vi "TEMPDo.vi"(8 "error in (no error)":errorcluster, 10 "Actor in":refnum<class "Actor.lvclass">, 11 "DNL_Message Template":refnum<class "Message.lvclass">) -> (0 "error out":errorcluster, 2 "Actor out":refnum<class "Actor.lvclass">)   [LabVIEW 2016, in "AsynchReturn Template.lvclass"]
doc: "This VI delivers the message to the actor by calling the appropriate method(s) on the actor."
uses:
  AsynchReturn Template.lvclass
  <vilib>/ActorFramework/Actor/Actor.lvclass
  <vilib>/ActorFramework/Message/Message.lvclass
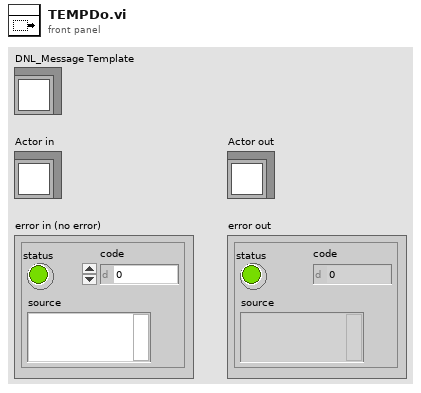
[diagram p1: front panel]
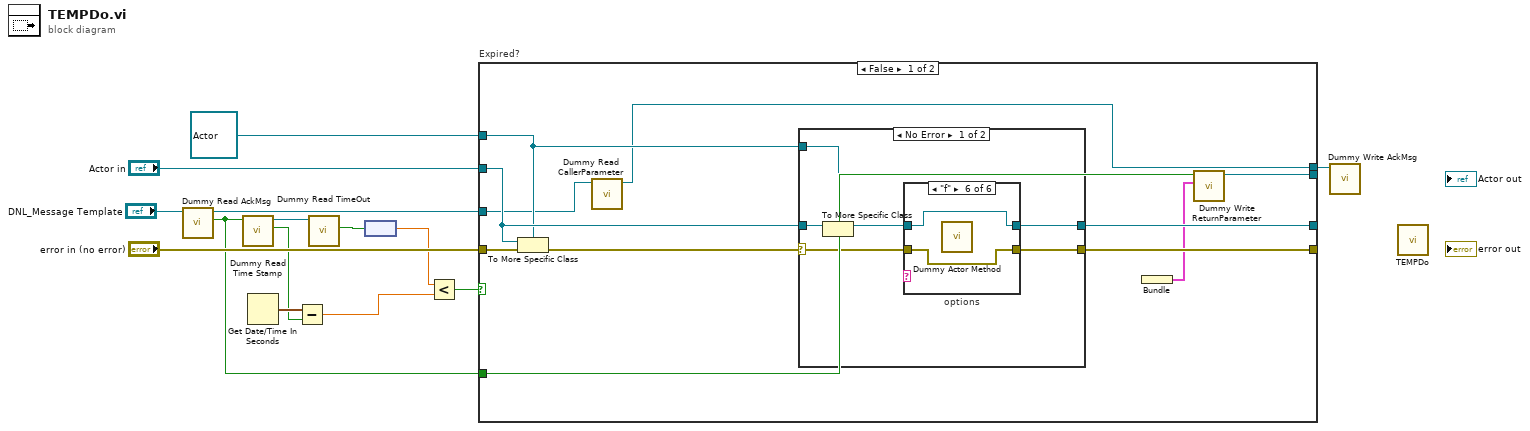
[diagram p0: block diagram]
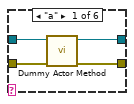
[diagram p2: hidden frame]
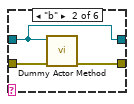
[diagram p3: hidden frame]
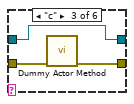
[diagram p4: hidden frame]
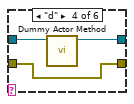
[diagram p5: hidden frame]
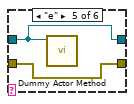
[diagram p6: hidden frame]
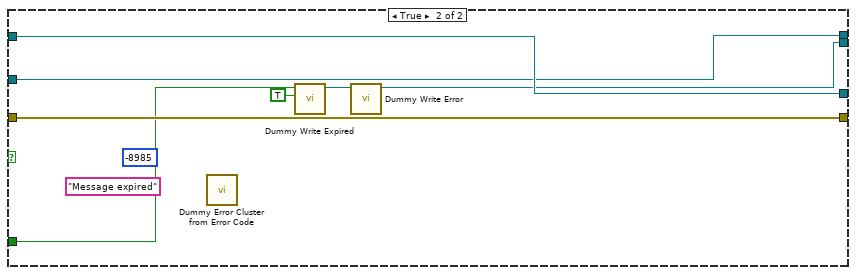
[diagram p8: hidden frame]
diagram:
  n1 = call "Dummy Read AckMsg.vi"("Actor in"="DNL_Message Template") -> ("Boolean"=w2:bool, "Actor out"=w3:refnum<class "Actor.lvclass">)  [unwired: 8 in, 1 out]
  n2 = call "Dummy Read Time Stamp.vi"("Actor in"=w2) -> ("Boolean"=w9:bool, "Actor out"=w8:refnum<class "Actor.lvclass">)  [unwired: 8 in, 1 out]
  n3 = Get Date/Time In Seconds() -> (seconds since 1Jan1904=w10:timestamp)
  n4 = Subtract(x=w10, y=w9) -> (x-y=w5:dbl)
  n5 = call "Dummy Read TimeOut.vi"("Actor in"=w8) -> ("Boolean"=w7:bool)  [unwired: 8 in, 2 out]
  n6 = node(w7) -> (w6:dbl[unit])
  n7 = Less?(x=w6, y=w5) -> (x < y?=w4:bool)
  n8 = case "Expired?" shown="False" w4 {
    tunnel: [w25 w56] -> _
    tunnel: [w24 w57] -> _
    tunnel: "Actor in" -> [w23 w57]
    tunnel: refnum<class "Actor.lvclass"> refnum ("Actor in") -> [w22 _]
    tunnel: "error in (no error)" -> [w21 w56]
    tunnel: w3 -> [w20 w52]
    tunnel: [w17 w52] -> w1
    tunnel: w2 -> [w18 w53]
    tunnel: [w16 w51] -> _
    frame False {
      n9 = To More Specific Class(target class=w22, reference=w23, error in=w21) -> (error out=w15:errorcluster)  [unwired: 1 out]
      n10 = call "Dummy Read CallerParameter.vi"("Actor in"=w20) -> ("Actor out"=w17:refnum<class "Actor.lvclass">)  [unwired: 8 in, 2 out]
      n11 = case "Error Case" shown="No Error" w15 {
        selector: w15 -> [w29 w50]
        tunnel: [w31 w50] -> w25
        tunnel: [w30 w49] -> w24
        tunnel: w23 -> [w28 w49]
        tunnel: w22 -> [w27 _]
        frame No Error {
          n12 = To More Specific Class(target class=w27, reference=w28) -> (specific class reference=w26:refnum<class "Actor.lvclass">)  [unwired: 1 in, 1 out]
          n13 = case "options" shown="\"f\"" {
            selector: _ -> [_ _ _ _ _ _]
            tunnel: [w35 w38 w41 w44 w45 w47] -> w31
            tunnel: [w34 w36 w39 w42 w46 w48] -> w30
            tunnel: w29 -> [w33 w37 w40 w44 w45 w47]
            tunnel: w26 -> [w32 w36 w39 w43 w46 w48]
            frame "a" {
              n14 = call "Dummy Actor Method.vi"("error in (no error)"=w33, "Actor in"=w32) -> ("error out"=w35:errorcluster, "Actor out"=w34:refnum<class "Actor.lvclass">)  [unwired: 8 in]
            }
            frame "b" {
              n15 = call "Dummy Actor Method.vi"("error in (no error)"=w37, "Actor in"=w36) -> ("error out"=w38:errorcluster)  [unwired: 8 in, 1 out]
            }
            frame "c" {
              n16 = call "Dummy Actor Method.vi"("error in (no error)"=w40) -> ("error out"=w41:errorcluster)  [unwired: 9 in, 1 out]
            }
            frame "d" {
              n17 = call "Dummy Actor Method.vi"("Actor in"=w43) -> ("Actor out"=w42:refnum<class "Actor.lvclass">)  [unwired: 9 in, 1 out]
            }
            frame "e" {
              n18 = call "Dummy Actor Method.vi"("Actor in"=w46) -> ()  [unwired: 9 in, 2 out]
            }
            frame "f" {
              n19 = call "Dummy Actor Method.vi"() -> ()  [unwired: 10 in, 2 out]
            }
          }
        }
        frame Error {
        }
      }
      n20 = Bundle ("Out-Bundler")() -> (w19:cluster{void})  [unwired: 2 in]
      n21 = call "Dummy Write ReturnParameter.vi"("Boolean"=w19, "Actor in"=w18) -> ("Actor out"=w16:refnum<class "Actor.lvclass">)  [unwired: 7 in, 1 out]
    }
    frame True {
      (unwired) -8985 ("ErrorCode")
      (unwired) "Message expired" ("ErrorMsg")
      n22 = call "Dummy Error Cluster from Error Code.vi"() -> ()  [unwired: 9 in, 3 out]
      n23 = call "Dummy Write Expired.vi"("Boolean"=TRUE, "Actor in"=w53) -> ("Actor out"=w55:refnum<class "Actor.lvclass">)  [unwired: 7 in, 1 out]
      n24 = call "Dummy Write Error.vi"("Actor in"=w55) -> ("Actor out"=w51:refnum<class "Actor.lvclass">)  [unwired: 8 in, 1 out]
    }
  }
  n25 = call "Dummy Write AckMsg.vi"("Actor in"=w1) -> ()  [unwired: 9 in, 2 out]
  n26 = call-parent "TEMPDo.vi"() -> ()  [unwired: 1 in]
